vi "AskChildToShow.vi"(8 "error in (no error)":errorcluster, 11 "loop data in":T1) -> (0 "error out":errorcluster, 3 "loop data out":T1)   [LabVIEW 2021, in "TipStripOOPanel.lvlib"]
uses:
  TipStripOOPanel.lvlib
  Loop Data Parent.ctl
  Classes/TipPanel/TipPanel.lvclass
  C:/Program Files/National Instruments/LabVIEW 2021/vi.lib/IlluminatedG/IG OOPanel/OOPanel/Panel/Panel.lvclass
  <vilib>/IlluminatedG/IG OOPanel/OOPanel/Manager/Manager.lvclass
  PanelMap.ctl
  PanelMapData.ctl
  Classes/TipPanel/ToPanelUEWrapper.ctl
  Classes/TipPanel/ToPanelUE.ctl
  <vilib>/Futures/Futures/Promise/Promise.lvclass
  refs.ctl
  <vilib>/Utility/miscctls.llb/LVRectTypeDef.ctl
  <vilib>/Utility/miscctls.llb/LVBoundsTypeDef.ctl
  <vilib>/Utility/miscctls.llb/LVMapReplaceAction.ctl
  <vilib>/Futures/Futures/Futures.lvlib
  <vilib>/Futures/Futures/Future/Future.lvclass
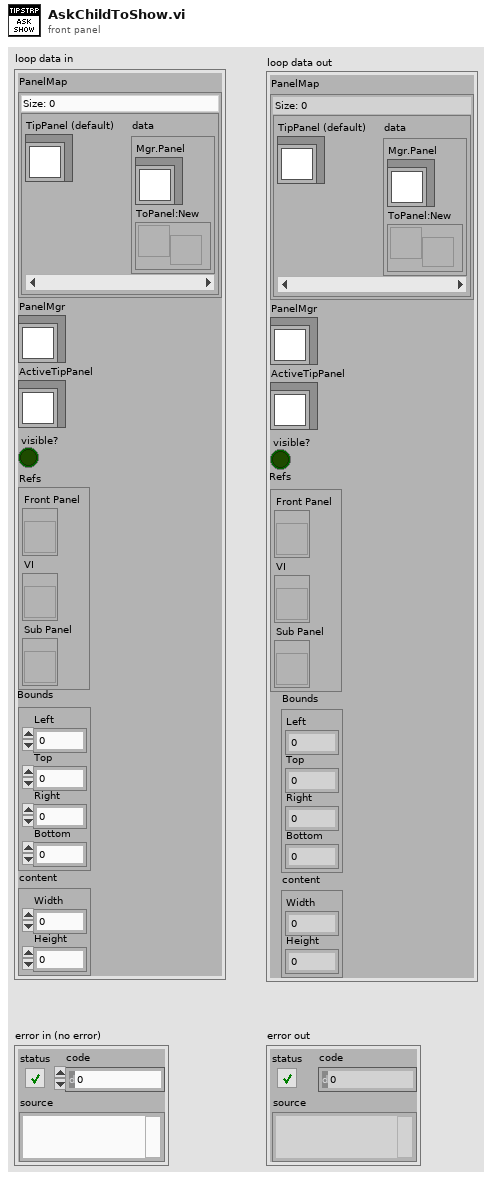
[diagram p1: front panel]
types:
  T1 = typedef "TipStripOOPanel.lvlib/Loop Data Parent.ctl" = cluster{"PanelMap":T2, "PanelMgr":refnum<class "Manager.lvclass">, "ActiveTipPanel":refnum<class "TipPanel.lvclass">, "visible?":bool, "Refs":T4, "Bounds":T5, "content":T6}
  T2 = typedef "TipStripOOPanel.lvlib/PanelMap.ctl" = map{refnum<class "TipPanel.lvclass">, T3}
  T3 = typedef "TipStripOOPanel.lvlib/PanelMapData.ctl" = cluster{"Mgr.Panel":refnum<class "TipPanel.lvclass">, "ToPanel:New":refnum<user-event>}
  T4 = typedef "TipStripOOPanel.lvlib/refs.ctl" = cluster{"Front Panel":refnum<vi>, "VI":refnum<vi>, "Sub Panel":refnum<vi>}
  T5 = typedef "LVRectTypeDef.ctl" = cluster{"Left":i16, "Top":i16, "Right":i16, "Bottom":i16}
  T6 = typedef "LVBoundsTypeDef.ctl" = cluster{"Width":u32, "Height":u32}
  T7 = typedef "TipStripOOPanel.lvlib/TipPanel.lvclass/ToPanelUEWrapper.ctl" = cluster{"NewPanel":T8}
  T8 = typedef "TipStripOOPanel.lvlib/TipPanel.lvclass/ToPanelUE.ctl" = cluster{"TipPanel":refnum<class>, "Promise.Size":refnum<class "Promise.lvclass">}
  T9 = typedef "LVMapReplaceAction.ctl" = enum32{"Modify Entry only if found", "Add or Modify Entry", "Delete Entry"}
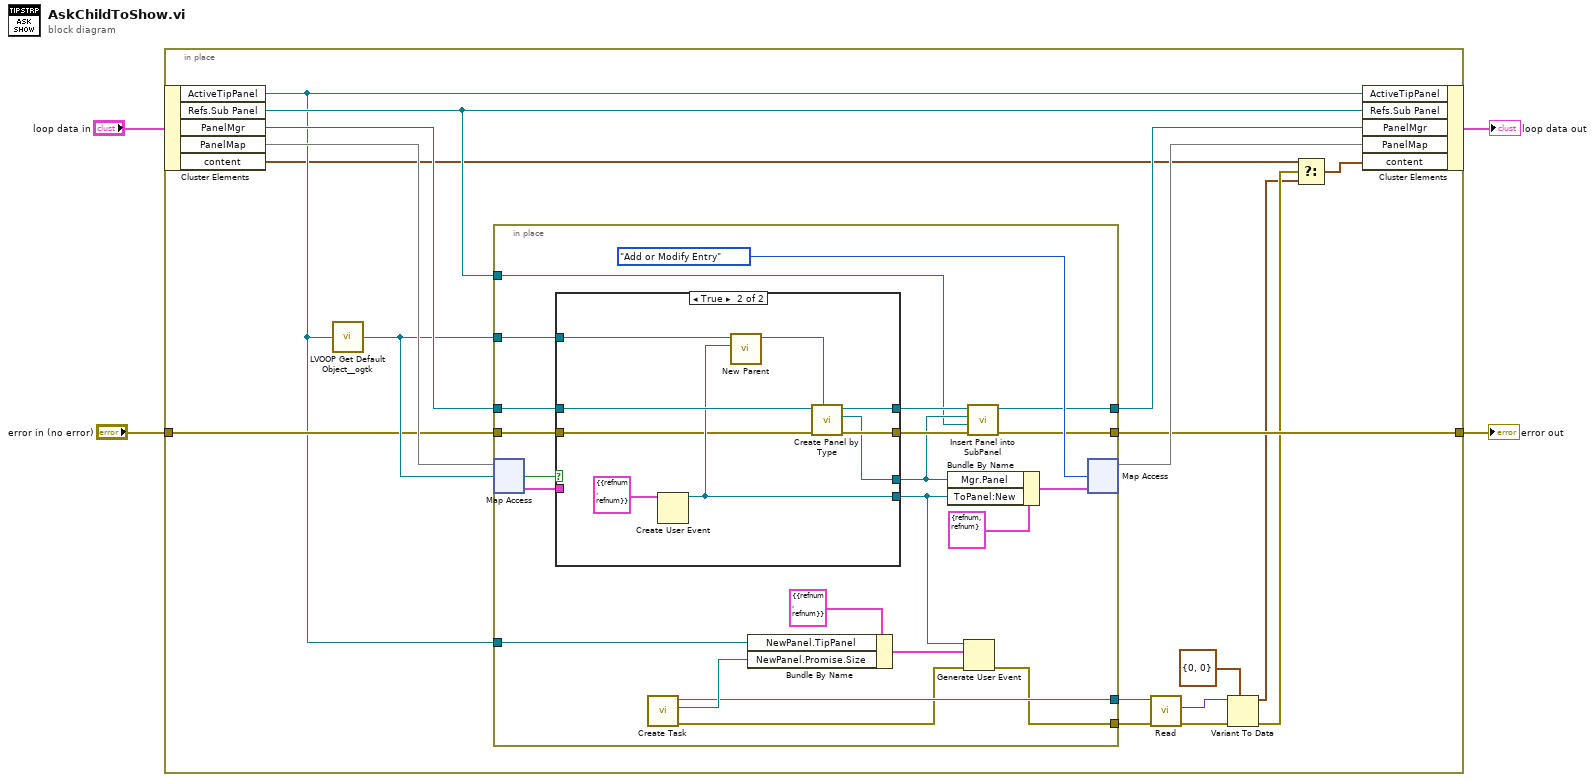
[diagram p0: block diagram]
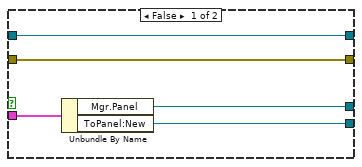
[diagram p2: hidden frame]
diagram:
  n1 = in-place {
    in-place-border: "error in (no error)" -> [w17]
    in-place-border: [w15] -> w1
    n2 = in-place-cluster #1("loop data in") -> ("ActiveTipPanel"=w14:refnum<class "TipPanel.lvclass">, "Refs.Sub Panel"=w16:refnum<vi>, "PanelMgr"=w20:refnum<class "Manager.lvclass">, "PanelMap"=w22:T2, "content"=w5:T6)
    n3 = call <userlib>:"LVOOP Get Default Object__ogtk.vi"("Object"=w14) -> ("Object Default Instance"=w18:refnum<class "TipPanel.lvclass">)
    n4 = in-place {
      in-place-border: w20 -> [w41]
      in-place-border: [w33] -> w19
      in-place-border: w18 -> [w40]
      in-place-border: w17 -> [w39]
      in-place-border: w14 -> [w29]
      in-place-border: w16 -> [w23]
      in-place-border: [w31] -> w15
      in-place-border: [w26] -> w13
      in-place-border: [w25] -> w9
      n5 = in-place-map #2(w22, w18) -> (w42:T3, w44:bool)  [unwired: 1 in]
      n6 = case shown="True" w44 {
        tunnel: w42 -> [w47 _]
        tunnel: w41 -> [w49 w58]
        tunnel: [w49 w57] -> w35
        tunnel: w40 -> [_ w56]
        tunnel: [w48 w54] -> w34
        tunnel: w39 -> [w48 w50]
        tunnel: [w45 w53] -> w32
        tunnel: [w46 w52] -> w36
        frame False {
          n7 = Unbundle By Name(w47) -> ("Mgr.Panel"=w45:refnum<class "TipPanel.lvclass">, "ToPanel:New"=w46:refnum<user-event>)
        }
        frame True {
          n8 = Create User Event(user event datatype=T7 {"NewPanel"={"TipPanel"=refnum, "Promise.Size"=refnum}} ("Cluster")) -> (user event=w52:refnum<user-event>)  [unwired: 1 in, 1 out]
          n9 = call "New Parent.vi"("ToPanel:New"=w52, "TipPanel in"=w56) -> ("TipPanel out"=w55:refnum<class "TipPanel.lvclass">)  [unwired: 8 in, 1 out]
          n10 = call <vilib>:"Create Panel by Type.vi"("Panel Type"=w55, "error in (no error)"=w50, "Manager in"=w58) -> ("error out"=w54:errorcluster, "Panel"=w53:refnum<class "TipPanel.lvclass">, "Manager out"=w57:refnum<class "Manager.lvclass">)  [unwired: 6 in]
        }
      }
      n11 = call <vilib>:"Create Task.vi"() -> ("error out"=w24:errorcluster, "Promise out"=w27:refnum<class "Promise.lvclass">, "Future out"=w26:refnum<class "Future.lvclass">)  [unwired: 9 in]
      n12 = Bundle By Name(cluster=T7 {"NewPanel"={"TipPanel"=refnum, "Promise.Size"=refnum}} ("Cluster"), "NewPanel.TipPanel"=w29, "NewPanel.Promise.Size"=w27) -> (w28:T7)
      n13 = Bundle By Name(cluster=T3 {"Mgr.Panel"=refnum, "ToPanel:New"=refnum} ("data"), "Mgr.Panel"=w32, "ToPanel:New"=w36) -> (w37:T3)
      n14 = Generate User Event(user event=w36, event data cluster=w28, error in=w24) -> (error out=w25:errorcluster)  [unwired: 1 in, 1 out]
      n15 = call <vilib>:"Insert Panel into SubPanel.vi"("error in (no error)"=w34, "SubPanel"=w23, "Panel In"=w32, "Manager in"=w35) -> ("error out"=w31:errorcluster, "Manager out"=w33:refnum<class "Manager.lvclass">)  [unwired: 5 in, 1 out]
      n16 = in-place-map #2(w37, LVMapReplaceAction."Add or Modify Entry" ("action")) -> (w21:T2)  [unwired: 2 out]
    }
    n17 = call <vilib>:"Read.vi"("error in (no error)"=w9, "Future in"=w13) -> ("error out"=w11:errorcluster, "Result value"=w12:variant)  [unwired: 6 in, 2 out]
    n18 = Variant To Data(error in=w11, type=T6 {"Width"=0, "Height"=0} ("content size"), Variant=w12) -> (data=w7:T6, error out=w8:errorcluster)
    n19 = Select(t=w5, s=w8, f=w7) -> (s? t:f=w6:T6)
    n20 = in-place-cluster #1("ActiveTipPanel"=w14, "Refs.Sub Panel"=w16, "PanelMgr"=w19, "PanelMap"=w21, "content"=w6) -> (→"loop data out":T1)
  }
  "error out" <- w1
